vi "DrawCrossHairs.vi"(11 "Image In":T1) -> (3 "Image Out":T1)   [LabVIEW 2012]
uses:
  <vilib>/vision/Image Controls.llb/IMAQ Image.ctl
  <vilib>/vision/NI_Vision_Development_Module.lvlib
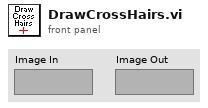
[diagram p1: front panel]
types:
  T1 = typedef "IMAQ Image.ctl" = refnum<image>
  T2 = cluster{"Red or Hue value":u8, "Green or Sat value":u8, "Blue or Luma or Val or Inten value":u8}
  T3 = cluster{dbl, "Blue or Luma or Val or Inten value":u8}
  T4 = cluster{"Blue or Luma or Val or Inten value":u8, dbl}
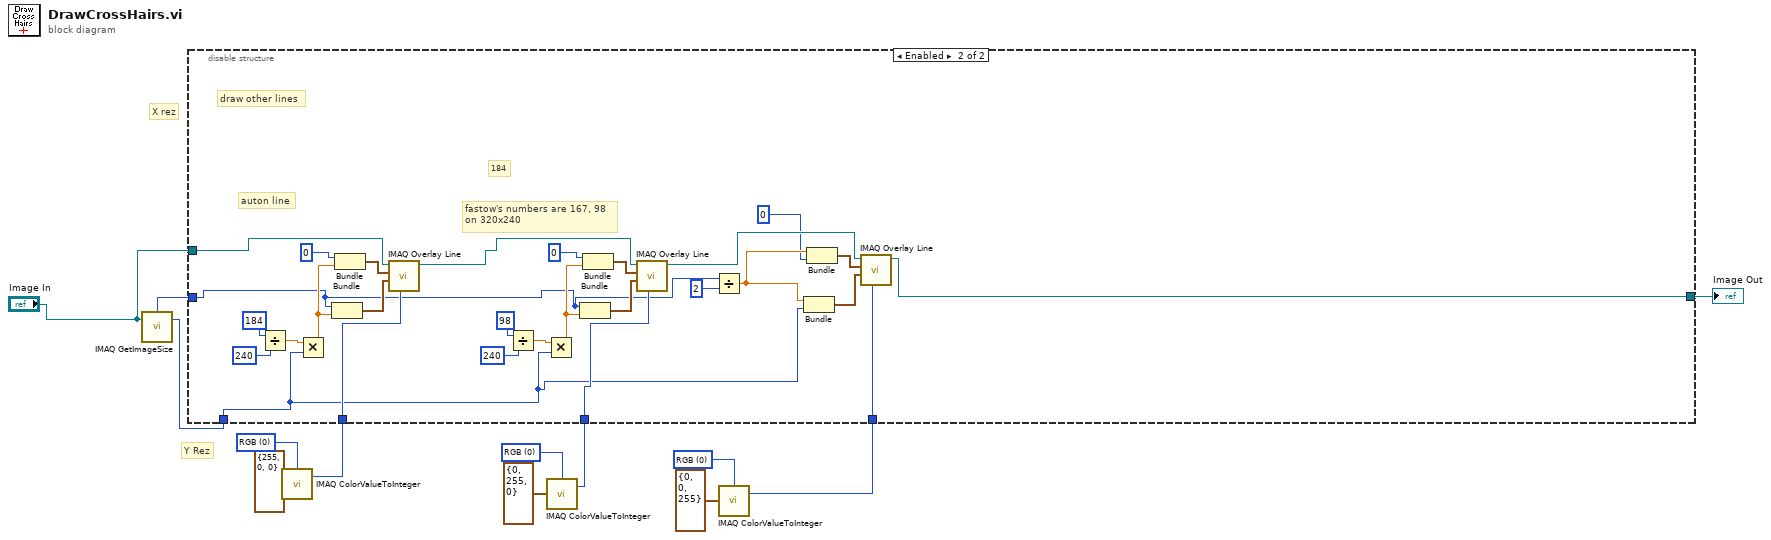
[diagram p0: block diagram]
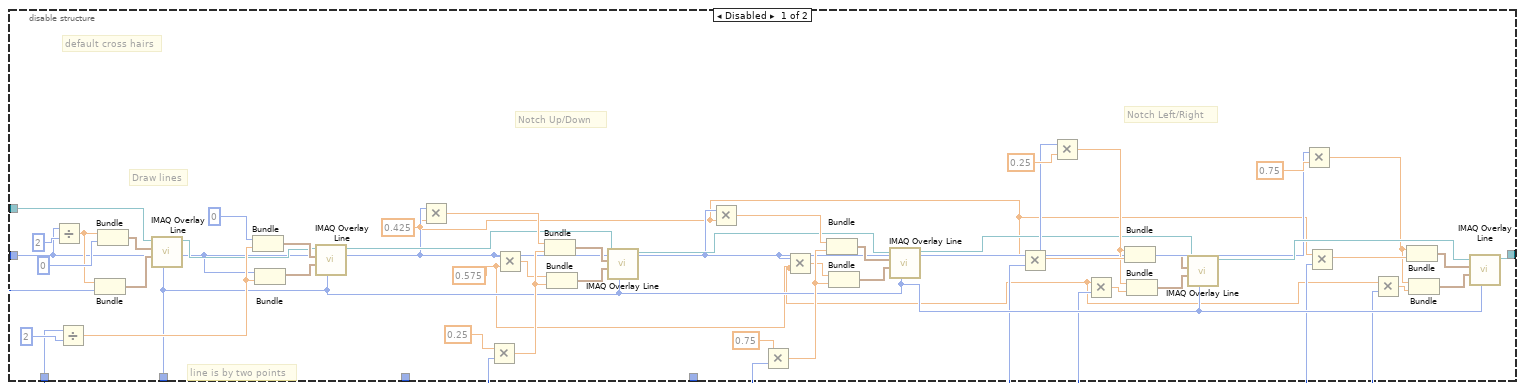
[diagram p2: hidden frame]
diagram:
  w2 = u16 0 items=["RGB", "HSL", "HSV", "HSI"] ("Color Mode")
  w7 = u16 0 items=["RGB", "HSL", "HSV", "HSI"] ("Color Mode")
  w13 = u16 0 items=["RGB", "HSL", "HSV", "HSI"] ("Color Mode")
  # "Y Rez"
  # "X rez"
  n1 = call "IMAQ GetImageSize"("Image"="Image In") -> ("Y Resolution"=w9:i32, "X Resolution"=w10:i32)  [unwired: 3 in, 1 out]
  n2 = call "IMAQ ColorValueToInteger"("Color Value"=T2 {"Red or Hue value"=255, "Green or Sat value"=0, "Blue or Luma or Val or Inten value"=0}, "Color Mode"=w13) -> ("U32 value"=w11:u32)  [unwired: 3 in, 3 out]
  n3 = call "IMAQ ColorValueToInteger"("Color Value"=T2 {"Red or Hue value"=0, "Green or Sat value"=255, "Blue or Luma or Val or Inten value"=0}, "Color Mode"=w7) -> ("U32 value"=w6:u32)  [unwired: 3 in, 3 out]
  n4 = call "IMAQ ColorValueToInteger"("Color Value"=T2 {"Red or Hue value"=0, "Green or Sat value"=0, "Blue or Luma or Val or Inten value"=255}, "Color Mode"=w2) -> ("U32 value"=w1:u32)  [unwired: 3 in, 3 out]
  n5 = disable-structure shown="Enabled" {
    disable-tunnel: "Image In" -> [w55 w82]
    disable-tunnel: w11 -> [w32 w79]
    disable-tunnel: w10 -> [w23 w64]
    disable-tunnel: w9 -> [w22 w60]
    disable-tunnel: [w16 w67] -> w8
    disable-tunnel: w6 -> [_ w71]
    disable-tunnel: w1 -> [_ w65]
    frame Disabled {
      w14 = 0.575
      w15 = 0.425
      # "default cross hairs"
      # "Notch Left/Right"
      # "Notch Up/Down"
      # "Draw lines"
      # "line is by two points"
      n6 = Divide(x=w23, y=2) -> (x/y=w54:dbl)
      n7 = Divide(x=w22, y=2) -> (x/y=w49:dbl)
      n8 = Bundle(w54, "Y Resolution"=w22) -> (w53:cluster{dbl, "Y Resolution":i32})  [unwired: 1 in]
      n9 = Bundle(w54, "Blue or Luma or Val or Inten value"=u8 0) -> (w56:T3)  [unwired: 1 in]
      n10 = call "IMAQ Overlay Line"("Color"=w32, "End Point"=w53, "Start Point"=w56, "Image"=w55) -> ("Image Out"=w48:T1)  [unwired: 6 in, 1 out]
      n11 = Bundle("Blue or Luma or Val or Inten value"=u8 0, w49) -> (w52:T4)  [unwired: 1 in]
      n12 = Bundle("X Resolution"=w23, w49) -> (w51:cluster{"X Resolution":i32, dbl})  [unwired: 1 in]
      n13 = call "IMAQ Overlay Line"("Color"=w32, "End Point"=w51, "Start Point"=w52, "Image"=w48) -> ("Image Out"=w39:T1)  [unwired: 6 in, 1 out]
      n14 = Multiply(x=w23, y=w15) -> (x*y=w42:dbl)
      n15 = Multiply(x=0.25, y=w22) -> (x*y=w44:dbl)
      n16 = Multiply(x=w23, y=w14) -> (x*y=w43:dbl)
      n17 = Bundle(w42, w44) -> (w41:cluster{dbl, dbl})  [unwired: 1 in]
      n18 = Bundle(w43, w44) -> (w40:cluster{dbl, dbl})  [unwired: 1 in]
      n19 = call "IMAQ Overlay Line"("Color"=w32, "End Point"=w40, "Start Point"=w41, "Image"=w39) -> ("Image Out"=w36:T1)  [unwired: 6 in, 1 out]
      n20 = Multiply(x=w23, y=w15) -> (x*y=w37:dbl)
      n21 = Multiply(x=0.75, y=w22) -> (x*y=w45:dbl)
      n22 = Multiply(x=w23, y=w14) -> (x*y=w38:dbl)
      n23 = Bundle(w37, w45) -> (w35:cluster{dbl, dbl})  [unwired: 1 in]
      n24 = Bundle(w38, w45) -> (w34:cluster{dbl, dbl})  [unwired: 1 in]
      n25 = call "IMAQ Overlay Line"("Color"=w32, "End Point"=w34, "Start Point"=w35, "Image"=w36) -> ("Image Out"=w17:T1)  [unwired: 6 in, 1 out]
      n26 = Multiply(x=w15, y=w22) -> (x*y=w25:dbl)
      n27 = Multiply(x=w23, y=0.25) -> (x*y=w24:dbl)
      n28 = Multiply(x=w14, y=w22) -> (x*y=w26:dbl)
      n29 = Bundle(w24, w25) -> (w21:cluster{dbl, dbl})  [unwired: 1 in]
      n30 = Bundle(w24, w26) -> (w20:cluster{dbl, dbl})  [unwired: 1 in]
      n31 = call "IMAQ Overlay Line"("Color"=w32, "End Point"=w20, "Start Point"=w21, "Image"=w17) -> ("Image Out"=w33:T1)  [unwired: 6 in, 1 out]
      n32 = Multiply(x=w23, y=0.75) -> (x*y=w27:dbl)
      n33 = Multiply(x=w15, y=w22) -> (x*y=w30:dbl)
      n34 = Multiply(x=w14, y=w22) -> (x*y=w31:dbl)
      n35 = Bundle(w27, w30) -> (w19:cluster{dbl, dbl})  [unwired: 1 in]
      n36 = Bundle(w27, w31) -> (w18:cluster{dbl, dbl})  [unwired: 1 in]
      n37 = call "IMAQ Overlay Line"("Color"=w32, "End Point"=w18, "Start Point"=w19, "Image"=w33) -> ("Image Out"=w16:T1)  [unwired: 6 in, 1 out]
    }
    frame Enabled {
      # "auton line"
      # "fastow's numbers are 167, 98\non 320x240"
      # "184"
      # "draw other lines"
      n38 = Divide(x=184 ("Numeric"), y=240) -> (x/y=w84:dbl)
      n39 = Multiply(x=w84, y=w60) -> (x*y=w83:dbl)
      n40 = Bundle("X Resolution"=w64, w83) -> (w80:cluster{"X Resolution":i32, dbl})  [unwired: 1 in]
      n41 = Bundle(0, w83) -> (w81:cluster{i32, dbl})  [unwired: 1 in]
      n42 = call "IMAQ Overlay Line"("Color"=w79, "End Point"=w80, "Start Point"=w81, "Image"=w82) -> ("Image Out"=w70:T1)  [unwired: 6 in, 1 out]
      n43 = Divide(x=98 ("Numeric"), y=240) -> (x/y=w75:dbl)
      n44 = Multiply(x=w75, y=w60) -> (x*y=w76:dbl)
      n45 = Bundle("X Resolution"=w64, w76) -> (w78:cluster{"X Resolution":i32, dbl})  [unwired: 1 in]
      n46 = Bundle(0, w76) -> (w77:cluster{i32, dbl})  [unwired: 1 in]
      n47 = call "IMAQ Overlay Line"("Color"=w71, "End Point"=w78, "Start Point"=w77, "Image"=w70) -> ("Image Out"=w66:T1)  [unwired: 6 in, 1 out]
      n48 = Divide(x=w64, y=2) -> (x/y=w62:dbl)
      n49 = Bundle(w62, "Y Resolution"=w60) -> (w68:cluster{dbl, "Y Resolution":i32})  [unwired: 1 in]
      n50 = Bundle(w62, 0) -> (w69:cluster{dbl, i32})  [unwired: 1 in]
      n51 = call "IMAQ Overlay Line"("Color"=w65, "End Point"=w68, "Start Point"=w69, "Image"=w66) -> ("Image Out"=w67:T1)  [unwired: 6 in, 1 out]
    }
  }
  "Image Out" <- w8
